vi "Reboot.vi"(7 "LabVIEW Web Service Request":refnum<class "Web Request.lvclass">) -> ()   [LabVIEW 2017]
uses:
  <vilib>/wsapi/Web Request.lvclass
  <vilib>/addons/Qbus/Qbus.lvclass
  <vilib>/addons/InsightCM/Devices/Shared/Common/Controller/Controller.lvlib
panel:
  out "error out":errorcluster
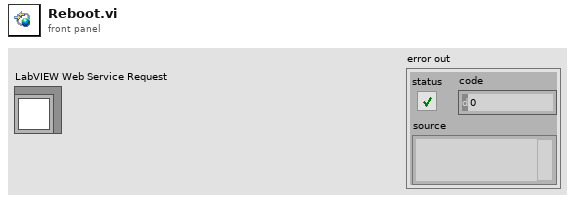
[diagram p1: front panel]
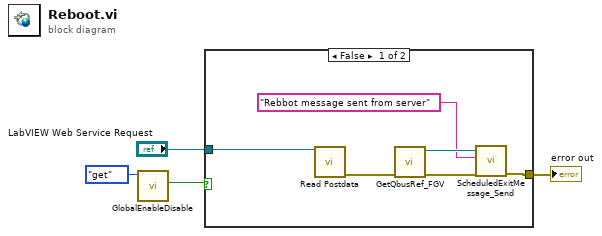
[diagram p0: block diagram]
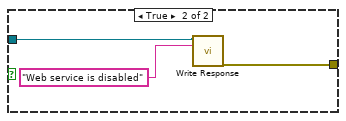
[diagram p2: hidden frame]
diagram:
  n1 = call "GlobalEnableDisable.vi"("action"=enum16{"init", "set", "get"}."get") -> ("DisableDeviceWebService"=w1:bool)  [unwired: 10 in]
  n2 = case shown="False" w1 {
    tunnel: "LabVIEW Web Service Request" -> [w10 w12]
    tunnel: [w7 w11] -> w3
    frame False {
      n3 = call <vilib>:"Read Postdata.vi"("LabVIEW Web Service Request"=w10) -> ("error out"=w9:errorcluster)  [unwired: 12 in, 2 out]
      n4 = call <vilib>:"GetQbusRef_FGV.vi"("error in (no error)"=w9) -> ("error out"=w8:errorcluster, "Qbus out"=w6:refnum<class "Qbus.lvclass">)  [unwired: 9 in]
      n5 = call <vilib>:"ScheduledExitMessage_Send.vi"("error in (no error)"=w8, "scheduled exit reason"="Rebbot message sent from server", "Qbus in"=w6) -> ("error out"=w7:errorcluster)  [unwired: 7 in, 1 out]
    }
    frame True {
      n6 = call <vilib>:"Write Response.vi"("LabVIEW Web Service Request"=w12, "response string"="Web service is disabled") -> ("error out"=w11:errorcluster)  [unwired: 12 in, 1 out]
    }
  }
  "error out" <- w3
